vi "Window-Time Series editor.vi"(9 "Standalone viewer?":bool=TRUE) -> ()   [LabVIEW 2020]
uses:
  User Interface/Visualisation/Timelapse Viewer/Typedefs/Custom slider-vertical.ctl
  User Interface/Visualisation/Timelapse Viewer/Typedefs/Time series viewer refs.ctl
  User Interface/Visualisation/Timelapse Viewer/Typedefs/Speed Viewer States enum.ctl
  <vilib>/Utility/miscctls.llb/LVPointTypeDef.ctl
  Typedefs/Save-Load enum.ctl
  <vilib>/vision/Image Controls.llb/IMAQ Image.ctl
  Typedefs/HW config states enum.ctl
  User Interface/Visualisation/Functional Imaging Viewer/Typedefs/Get-Set-Clear Control.ctl
  User Interface/Visualisation/Timelapse Viewer/Typedefs/Select Play-Stop button to show.ctl
  <vilib>/Utility/error.llb/DialogType.ctl
  User Interface/Visualisation/Timelapse Viewer/Cam video sync/Typedefs/Cam videos cluster.ctl
  User Interface/Visualisation/Timelapse Viewer/Globals/gl_Time series viewer globals.vi
  Global Variables/General Globals.vi
panel:
  out "Slider at frame #":i32 format="Slider at frame: %.0f"
  in  "Scrollbar":i32(c297)
  in  "Back":bool
  in  "Play":bool
  in  "Stop":bool
  in  "Tab Control":enum32{"Camera videos", "Speed data"}(tab)
  out "Cams":T2 {"Vid4 Rel time (ms)" format="%.0f ms"; "Vid3 Rel time (ms)" format="%.0f ms"; "Vid2 Rel time (ms)" format="%.0f ms"; "Vid1 Rel time (ms)" format="%.0f ms"}
  out "Actual number of speed points":i32 format="Actual of speed points: %.0f"
  out "Speed Data":string[][](array[string])
  out "Expected speed values":dbl format="Expected speed points: %#_g"
  out "Original frame rate (fps)":dbl format="Original frame rate: %#.1f (fps)"
  out "Frame rate set (fps)":dbl format="Frame rate set: %#.1f (fps)"
  out "Actual frame rate (fps)":dbl format="Actual frame rate: %#.1f (fps)"
  out "AVI Mode ind":string="AVI mode:"
  out "Video length info":string="Duration: 00h 00m 00s, 0 frames"
  in  "AVI File Path":path
  out "Export images":bool
  out "Export snippet":bool
  in  "Selection sliders":cluster{i32, i32}(slide)={1, 5594} scale=1.0..3919.0
  out "Export vid":bool
  out "Stop (ind)":bool
  in  "Intensity":T3={0.0, 4095.0} scale=0.0..4095.0
  in  "Colour":enum16{"Gray", "Red", "Green"}(ring)
  out "Speed Graph":dbl[](graph) caption="Speed Chart"
  out "Image":T1(plugin-control)
  # "Date                         Time                  Time stamp           Speed (rpm)          Angle (deg)"
  # "Time series info"
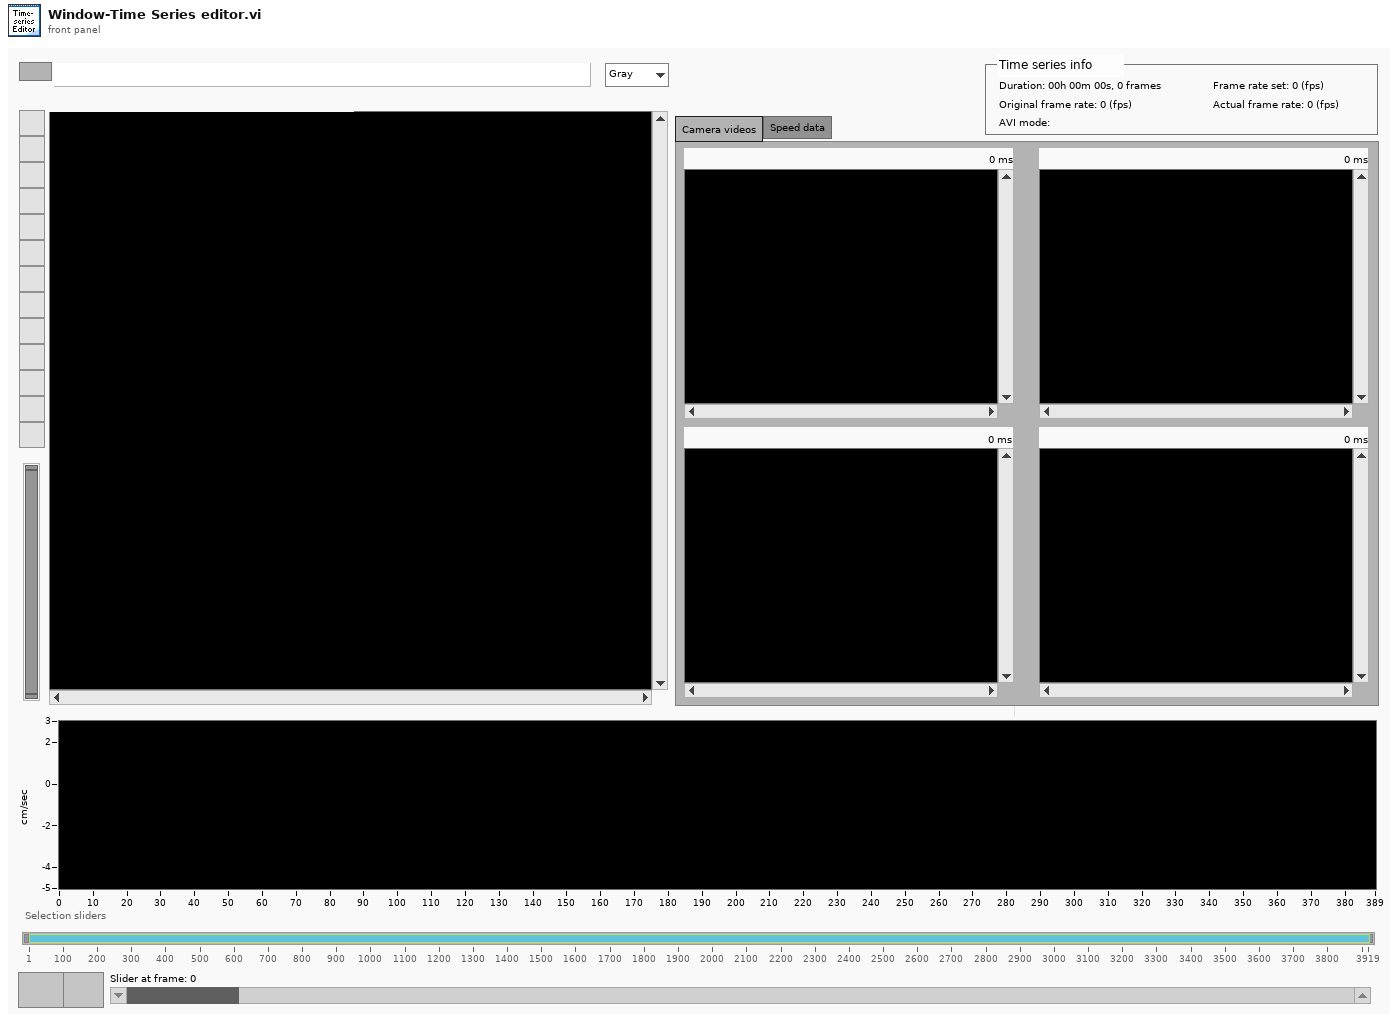
[diagram p1: front panel]
types:
  T1 = typedef "IMAQ Image.ctl" = refnum<image>
  T2 = cluster{"Vid 1":T1, "Vid 2":T1, "Vid 3":T1, "Vid 4":T1, "Vid1 Rel time (ms)":u32, "Vid2 Rel time (ms)":u32, "Vid3 Rel time (ms)":u32, "Vid4 Rel time (ms)":u32}
  T3 = typedef "Custom slider-vertical.ctl" = cluster{dbl, dbl}
  T4 = typedef "Time series viewer refs.ctl" = cluster{"This VI":refnum<vi>, "Image control":refnum<vi>, "AVI Mode ind":refnum<vi>, "Play":refnum<vi>, "Stop":refnum<vi>, "Back":refnum<vi>, "Scrollbar":refnum<vi>, "Video length info":refnum<vi>, "Expected speed values":refnum<vi>, "Intensity":refnum<vi>, "Path":refnum<vi>, "Selection sliders":refnum<vi>, "Speed Graph ref":refnum<vi>, "Frame rate set (fps)":refnum<vi>, "Number of rows to generate":refnum<vi>, "VL Image Array":refnum<vi>, "Image Scrollbar":refnum<vi>, "Channel to load":refnum<vi>, "Colour":refnum<vi>}
  T5 = typedef "Save-Load enum.ctl" = enum16{"Save to file", "Load from file", "Compare from file", "Save Backup"}
  T6 = enum16{"None", "Release queue", "Obtain queue", "Enqueue", "Get status", "Set status"}
  T7 = typedef "LVPointTypeDef.ctl" = cluster{"Horizontal":i16, "Vertical":i16}
  T8 = typedef "Speed Viewer States enum.ctl" = enum16{"Idle", "Initialise", "Playback", "Scroll bar event", "Speed cursor event", "Back to start", "Exit"}
  T9 = typedef "HW config states enum.ctl" = enum16{"Load from file", "Save to file", "Save backup", "Write all", "Read all", "Write XY stage settings", "Write DAQ FPGA settings", "Write Control FPGA settings", "Write Phys Channels", "Write System Config", "Write HW Config", "Save System Config", "Save HW Config", "Clear", "Compare from file"}
  T10 = typedef "Image Type" = u32
  T11 = typedef "Custom slider-horisontal.ctl" = cluster{dbl, dbl}
  T12 = typedef "Get-Set-Clear Control.ctl" = enum16{"Get", "Set", "Clear"}
  T13 = typedef "Select Play-Stop button to show.ctl" = enum16{"Show Play button", "Show Stop button"}
  T14 = typedef "Cam videos cluster.ctl" = cluster{"Vid 1":T1, "Vid 2":T1, "Vid 3":T1, "Vid 4":T1, "Vid1 Rel time (ms)":u32, "Vid2 Rel time (ms)":u32, "Vid3 Rel time (ms)":u32, "Vid4 Rel time (ms)":u32}
  T15 = typedef "DialogType.ctl" = u16
  T16 = typedef "AVI modes refs cluster.ctl" = cluster{"AVI1 ref":T17, "AVI2 refs":T18[], "AVI # frames":u32[]}
  T17 = typedef "AviRefnum.ctl" = refnum<k1>
  T18 = typedef "IMAQ AVI2 Refnum.ctl" = refnum<k20>
  T19 = cluster{"Start Frame No":i32, "End Frame No":i32}
  T20 = typedef "AVI implementation enum.ctl" = enum16{"AVI1", "AVI2"}
  T21 = cluster{"# of frames to export":i32, "Initial frame's owning file":T18, "8-bit AVI file path":path, "Cursors location":cluster{"Number of first frame":i32, "Number of last frame":i32}}
  T22 = enum32{"Invalid", "Standard", "Closed", "Hidden", "Minimized", "Maximized"}
  T23 = typedef "Speed graph behaviour enum.ctl" = enum16{"Scrolling data", "Scrolling cursor"}
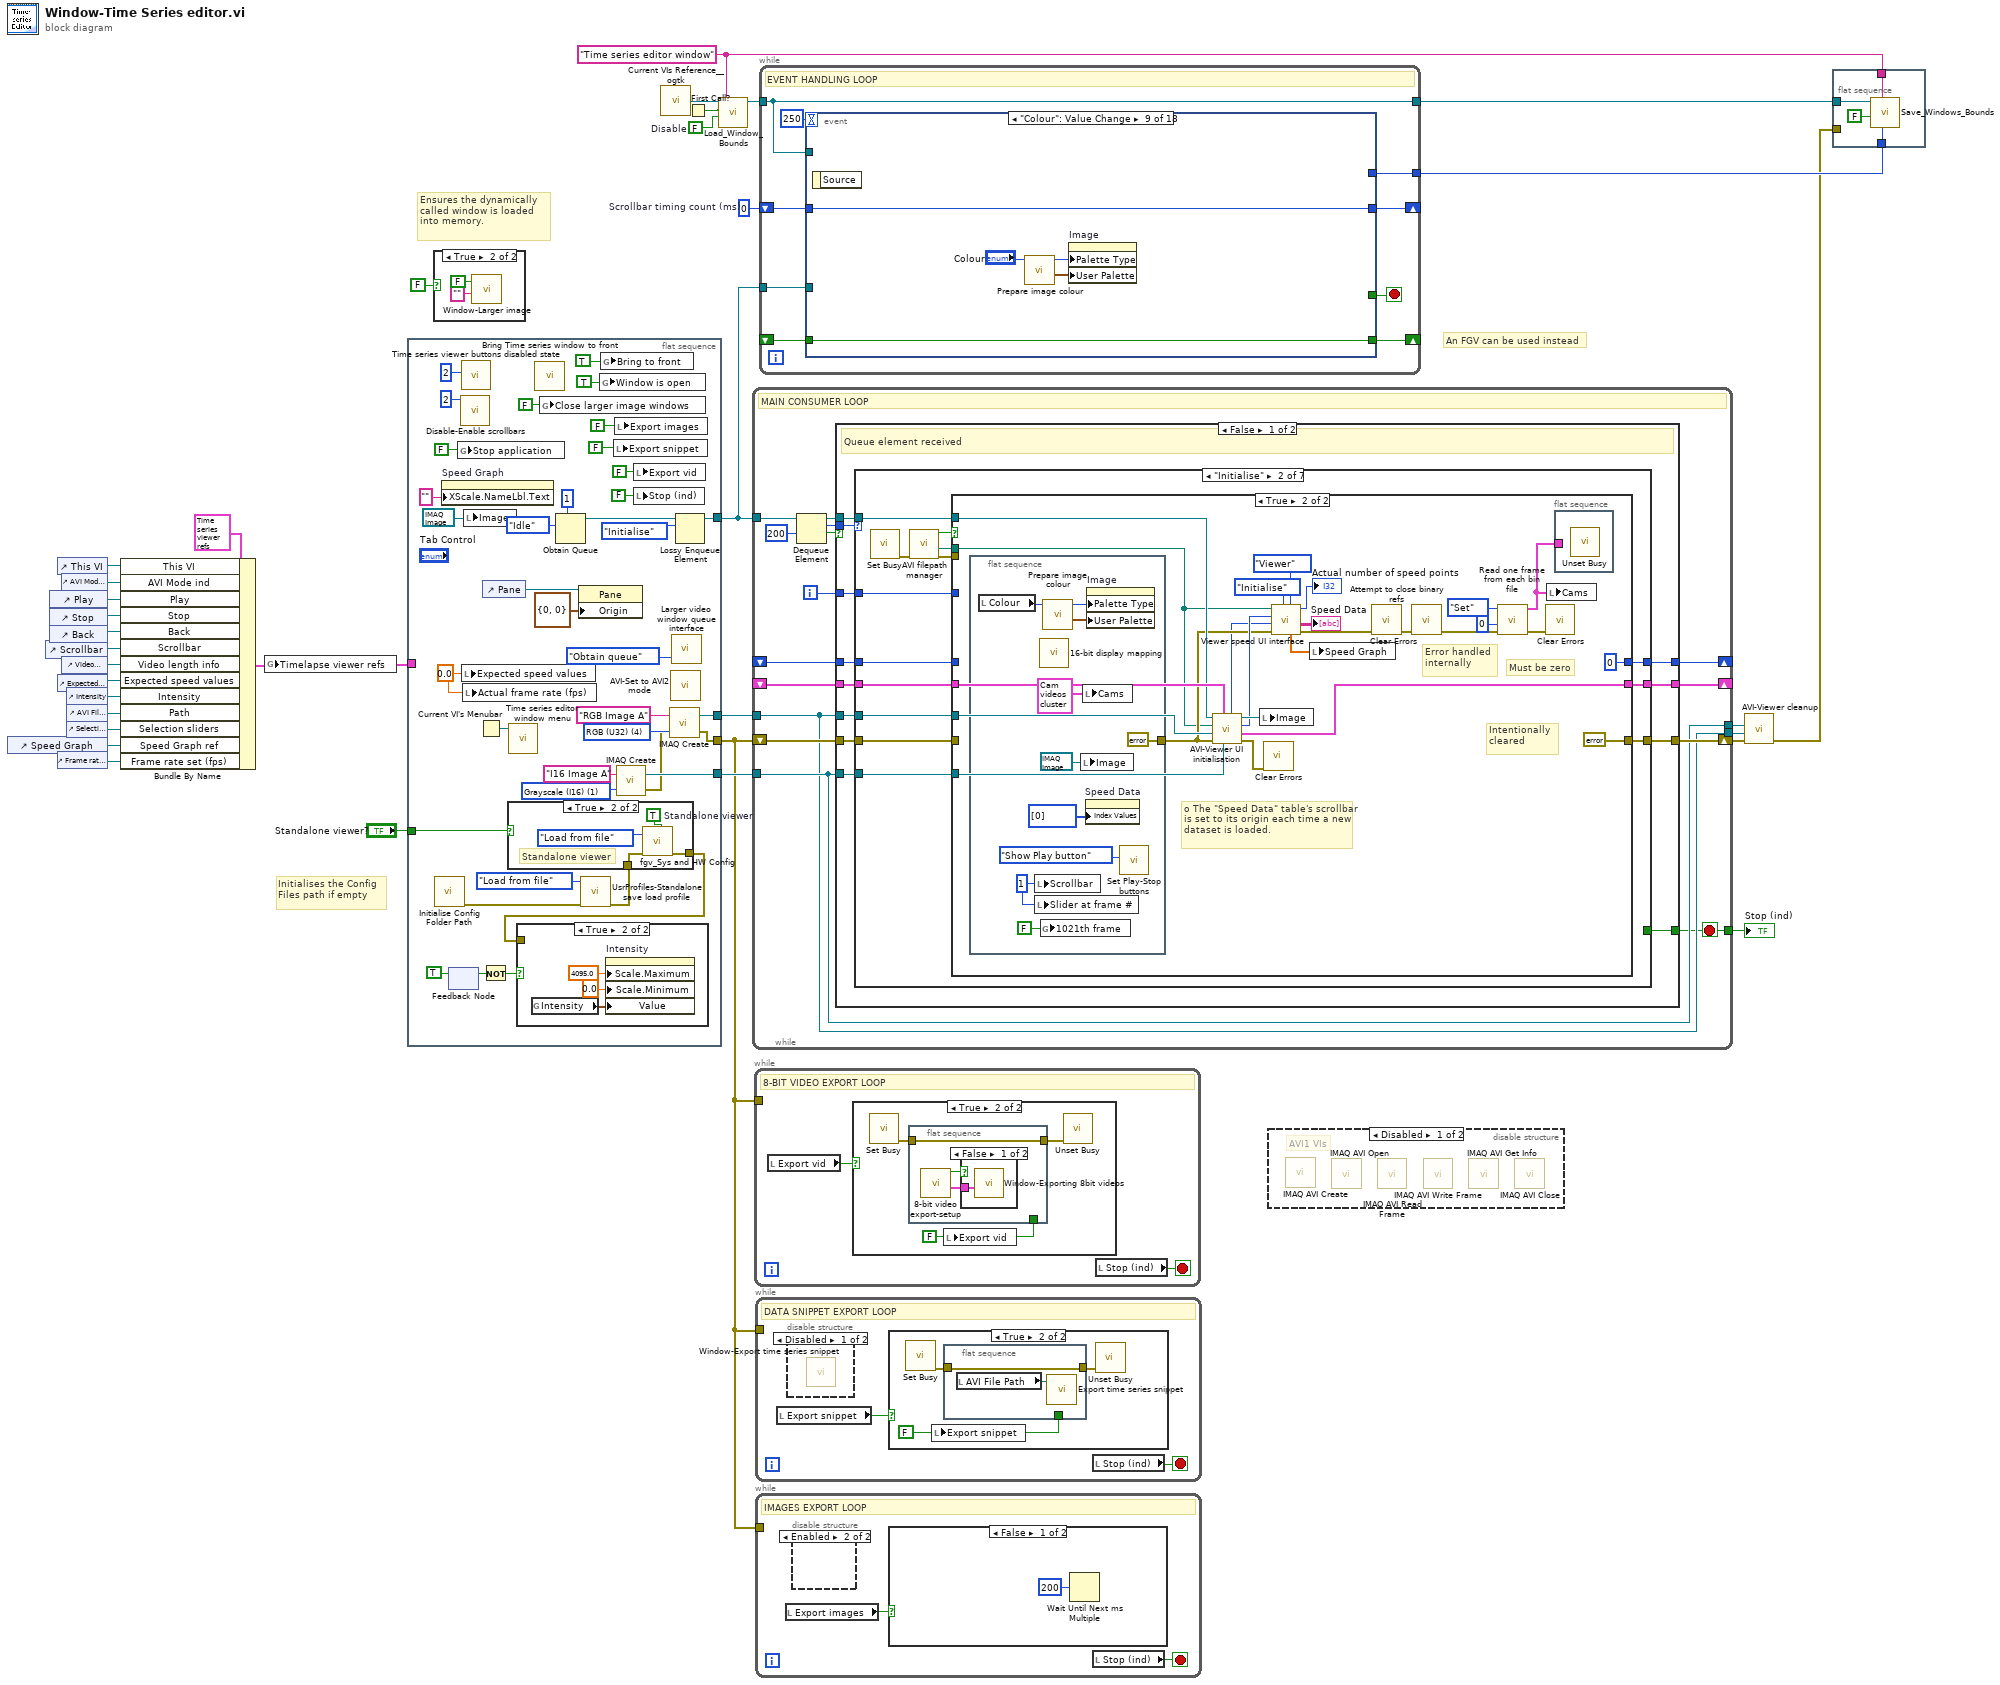
[diagram p0: block diagram]
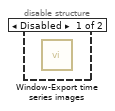
[diagram p3: hidden frame]
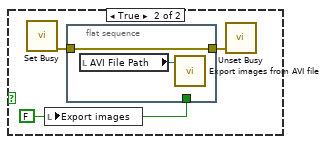
[diagram p4: hidden frame]
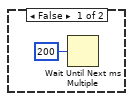
[diagram p6: hidden frame]
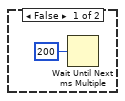
[diagram p8: hidden frame]
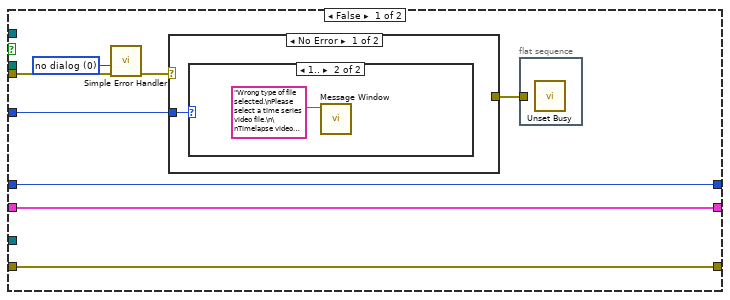
[diagram p13: hidden frame]
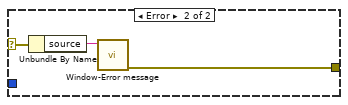
[diagram p15: hidden frame]
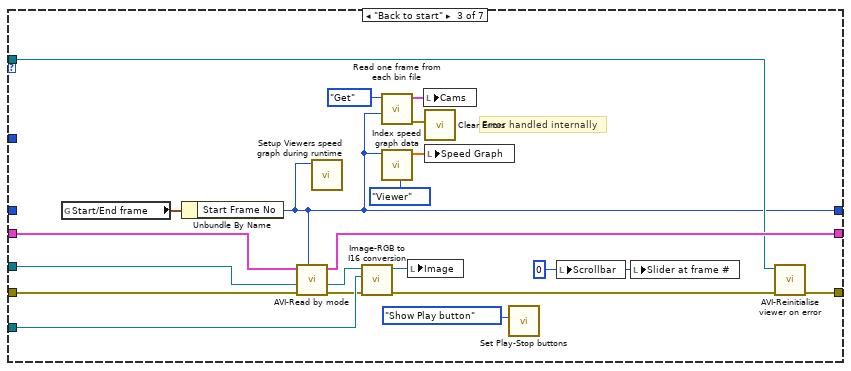
[diagram p16: hidden frame]
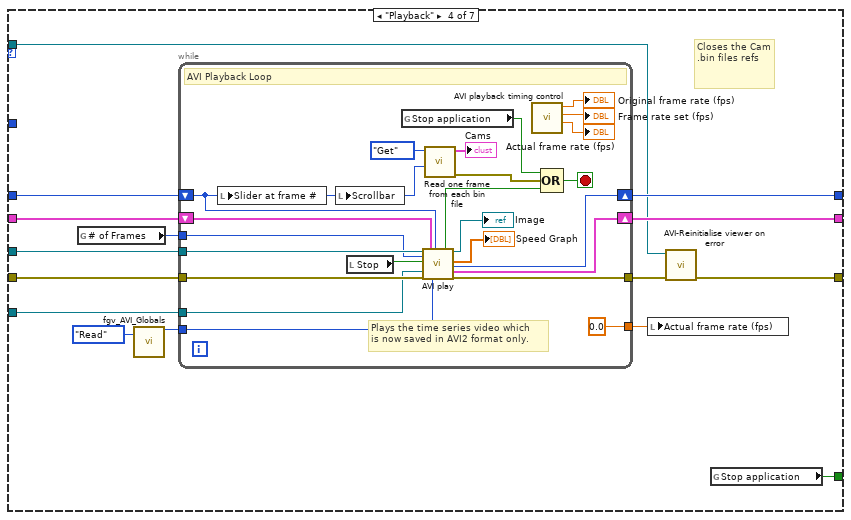
[diagram p17: hidden frame]
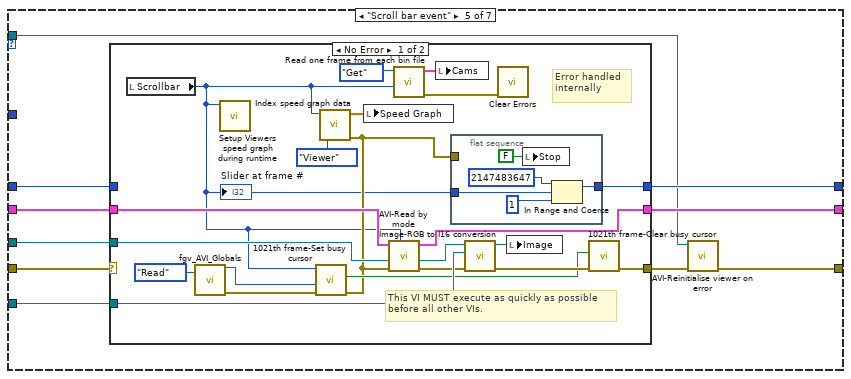
[diagram p18: hidden frame]
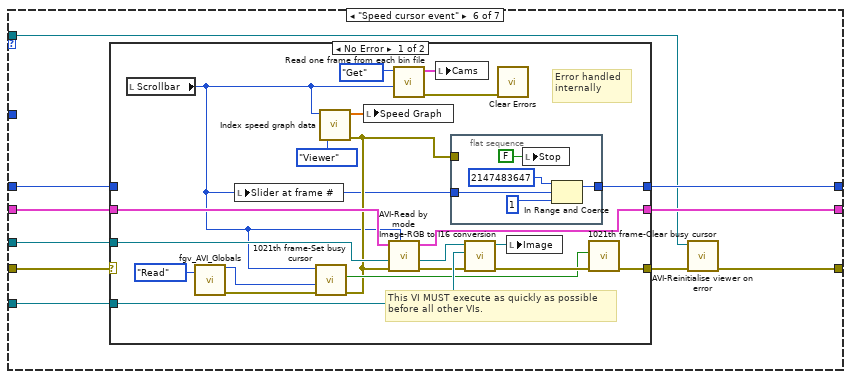
[diagram p20: hidden frame]
diagram:
  w9 = FALSE  # Disable
  w8 = "Time series editor window" ("Window Name (i.e. Key)")
  w20 = u32 0  # Scrollbar timing count (ms)
  # "Initialises the Config Files path if empty"
  # "Ensures the dynamically called window is loaded into memory."
  # "An FGV can be used instead"
  n1 = control-ref of="Speed Graph"() -> (w13:refnum<vi>)
  n2 = control-ref of="Scrollbar"() -> (w24:refnum<vi>)
  n3 = control-ref of="Play"() -> (w27:refnum<vi>)
  n4 = control-ref of="Stop"() -> (w26:refnum<vi>)
  n5 = control-ref of="Back"() -> (w25:refnum<vi>)
  n6 = control-ref of="This VI"() -> (w17:refnum<vi>)
  n7 = control-ref of="Expected speed values"() -> (w22:refnum<vi>)
  n8 = control-ref of="Frame rate set (fps)"() -> (w2:refnum<vi>)
  n9 = control-ref of="AVI Mode ind"() -> (w30:refnum<vi>)
  n10 = control-ref of="Video length info"() -> (w23:refnum<vi>)
  n11 = control-ref of="Intensity"() -> (w21:refnum<vi>)
  n12 = control-ref of="AVI File Path"() -> (w19:refnum<vi>)
  n13 = control-ref of="Selection sliders"() -> (w14:refnum<vi>)
  n14 = Bundle By Name(cluster=T4 {"This VI"=refnum, "Image control"=refnum, "AVI Mode ind"=refnum, "Play"=refnum, "Stop"=refnum, "Back"=refnum, "Scrollbar"=refnum, "Video length info"=refnum, "Expected speed values"=refnum, "Intensity"=refnum, "Path"=refnum, "Selection sliders"=refnum, "Speed Graph ref"=refnum, "Frame rate set (fps)"=refnum, "Number of rows to generate"=refnum, "VL Image Array"=refnum, "Image Scrollbar"=refnum, "Channel to load"=refnum, "Colour"=refnum}, "This VI"=w17, "AVI Mode ind"=w30, "Play"=w27, "Stop"=w26, "Back"=w25, "Scrollbar"=w24, "Video length info"=w23, "Expected speed values"=w22, "Intensity"=w21, "Path"=w19, "Selection sliders"=w14, "Speed Graph ref"=w13, "Frame rate set (fps)"=w2) -> (w16:T4)
  n15 = global write "gl_Time series viewer globals.vi" "Timelapse viewer refs"(w16) -> ()
  n16 = flat-sequence {
    tunnel: [w70] -> w34
    tunnel: [w67] -> w33
    tunnel: [w60] -> w12
    tunnel: [w63] -> w31
    tunnel: w16 -> [_]
    tunnel: "Standalone viewer?" -> [w35]
    frame #0 {
      w57 = 0.0 ("Expected speed points")
      w69 = T10 1 items=["Grayscale (U8)", "Grayscale (I16)", "Grayscale (SGL)", "Complex (CSG)", "RGB (U32)", "HSL (U32)", "RGB (U64)", "Grayscale (U16)"] ("Image Type")
      w71 = T10 4 items=["Grayscale (U8)", "Grayscale (I16)", "Grayscale (SGL)", "Complex (CSG)", "RGB (U32)", "HSL (U32)", "RGB (U64)", "Grayscale (U16)"] ("Image Type")
      n17 = call "Initialise Config Folder Path.vi"() -> ("error out"=w42:errorcluster)  [unwired: 9 in, 2 out]
      n18 = property on="Speed Graph" class="WFGraph (strict)"("XScale.NameLbl.Text"="" ("X Scale.Name Label.Text")) -> ()  [unwired: 2 in, 2 out]
      n19 = feedback #1() -> (w38:bool)  [unwired: 1 in]
      n20 = feedback-in #1(TRUE) -> ()
      n21 = global write "General Globals.vi" "Stop application"(FALSE ("Stop application")) -> ()
      n22 = call "Disable-Enable scrollbars.vi"("Disabled state"=2) -> ()  [unwired: 10 in, 1 out]
      n23 = call "Time series viewer buttons disabled state.vi"("Disabled"=2) -> ()  [unwired: 10 in, 1 out]
      n24 = local write "Expected speed values"(w57) -> ()
      n25 = local write "Actual frame rate (fps)"(w57) -> ()
      n26 = local write "Image"(T1 refnum ("Image")) -> ()
      n27 = Current VI's Menubar() -> (w56:refnum<k9>)
      n28 = Not(x=w38) -> (.not. x?=w40:bool)
      n29 = control-ref of="Pane"() -> (w58:refnum<vi>)
      n30 = call "Time series editor window menu.vi"("menu"=w56) -> ()  [unwired: 9 in, 2 out]
      n31 = call "Bring Time series window to front.vi"() -> ()  [unwired: 12 in]
      n32 = global write "gl_Time series viewer globals.vi" "Close larger image windows"(FALSE ("Close larger image window")) -> ()
      n33 = Obtain Queue(max queue size (-1, unlimited)=1, element data type=Speed_Viewer_States_enum."Idle" ("States")) -> (queue out=w64:refnum<queue>)  [unwired: 3 in, 2 out]
      n34 = property class="Pane"(reference=w58, "Origin"=T7 {"Horizontal"=0, "Vertical"=0}) -> ()  [unwired: 1 in, 2 out]
      n35 = call "UsrProfiles-Standalone save load profile.vi"("Error in"=w42, "Function"=Save-Load_enum."Load from file") -> ("error out"=w37:errorcluster)  [unwired: 9 in]
      n36 = case shown="True" w35 {
        tunnel: w37 -> [w73 w76]
        tunnel: [w73 w75] -> w36
        frame False {
          # "No need to load the system\nconfig. Already loaded."
        }
        frame True {
          w74 = TRUE  # Standalone viewer
          # "Standalone viewer"
          n37 = call "fgv_Sys and HW Config.vi"("Standalone viewer initialisation?"=w74, "Function"=HW_config_states_enum."Load from file", "error in (no error)"=w76) -> ("error out"=w75:errorcluster)  [unwired: 6 in, 2 out]
        }
      }
      n38 = case shown="True" w40 {
        tunnel: w36 -> [_ _]
        frame False {
        }
        frame True {
          n39 = global read "gl_Time series viewer globals.vi" "Intensity"() -> (w78:T11)
          n40 = property on="Intensity" class="Slide (strict)"("Scale.Maximum"=4095.0 ("Scale.Range:Maximum"), "Scale.Minimum"=0.0 ("Scale.Range:Minimum"), "Value"=w78) -> ()  [unwired: 2 in, 2 out]
        }
      }
      n41 = global write "gl_Time series viewer globals.vi" "Window is open"(TRUE ("Window is open")) -> ()
      n42 = global write "gl_Time series viewer globals.vi" "Bring to front"(TRUE ("Bring Timelapse Editor to front")) -> ()
      n43 = local write "Export snippet"(FALSE ("Export data subset")) -> ()
      n44 = local write "Export images"(FALSE ("Export data subset")) -> ()
      n45 = call "IMAQ Create"("Image Name"="I16 Image A", "Image Type"=w69) -> ("New Image"=w67:T1, "error out"=w61:errorcluster)  [unwired: 2 in, 1 out]
      n46 = local write "Export vid"(FALSE ("Export")) -> ()
      n47 = local write "Stop (ind)"(FALSE ("Boolean")) -> ()
      n48 = call "IMAQ Create"("Image Name"="RGB Image A", "Image Type"=w71, "error in (no error)"=w61) -> ("New Image"=w70:T1, "error out"=w60:errorcluster)  [unwired: 1 in, 1 out]
      n49 = call "AVI-Set to AVI2 mode.vi"() -> ()  [unwired: 11 in, 1 out]
      n50 = call "Larger video window queue interface.vi"("Function"=T6."Obtain queue") -> ()  [unwired: 10 in, 1 out]
      n51 = Lossy Enqueue Element(queue=w64, element=Speed_Viewer_States_enum."Initialise" ("States")) -> (queue out=w63:refnum<queue>)  [unwired: 1 in, 3 out]
    }
  }
  n52 = case shown="True" FALSE {
    frame False {
    }
    frame True {
      n53 = call "Window-Larger image.vi"("Image name"="", "Open maximised"=FALSE) -> ()  [unwired: 10 in]
    }
  }
  n54 = call <userlib>:"Current VIs Reference__ogtk.vi"() -> ("Current VI's reference"=w11:refnum<vi>)  [unwired: 5 in]
  n55 = First Call?() -> (First Call?: T/F=w10:bool)
  n56 = call "Load_Window_Bounds.vi"("Window Name (i.e. Key)"=w8, "Disable"=w9, "First Call"=w10, "Window VI's Ref"=w11) -> ("reference out"=w5:refnum<vi>)  [unwired: 4 in, 3 out]
  n57 = while {
    tunnel: w34 -> [w86]
    tunnel: w33 -> [w87]
    tunnel: [w87] -> w32
    shift-right: [w94] -> _
    shift-left: _ -> [w93]
    tunnel: w31 -> [w92]
    shift-right: [w88] -> _
    shift-left: _ -> [w97]
    tunnel: [w86] -> w18
    shift-right: [w95] -> w28
    shift-left: w12 -> [w96]
    tunnel: [w84] -> w15
    i -> [w83]
    stop <- w84 stop-if-true
    # "MAIN CONSUMER LOOP"
    n58 = Dequeue Element(queue=w92, timeout in ms (-1)=200) -> (queue out=w85:refnum<queue>, element=w89:T8, timed out?=w90:bool)  [unwired: 1 in, 1 out]
    n59 = case shown="False" w90 {
      tunnel: w97 -> [w109 w321]
      tunnel: [w108 w321] -> w88
      tunnel: w86 -> [w107 _]
      tunnel: w87 -> [w106 _]
      tunnel: w96 -> [w105 w320]
      tunnel: [w104 w320] -> w95
      tunnel: [w103 w322] -> w94
      tunnel: w93 -> [w102 w322]
      tunnel: w89 -> [w101 _]
      tunnel: [w100 w319] -> w84
      tunnel: w85 -> [w99 _]
      tunnel: w83 -> [w98 _]
      frame False {
        # "Queue element received"
        n60 = case shown="\"Initialise\"" w101 {
          tunnel: w109 -> [w111 w126 w192 w209 w238 w277 w313]
          tunnel: [w111 w122 w191 w203 w240 w279 w313] -> w108
          tunnel: w107 -> [_ w121 w189 w208 w239 w278 _]
          tunnel: w106 -> [_ w120 w190 w207 w242 w281 _]
          tunnel: w105 -> [w110 w124 w187 w206 w237 w276 w312]
          tunnel: [w110 w123 w182 w202 w235 w274 w311] -> w104
          tunnel: [w112 w125 w175 w205 w241 w280 1 ("Slide")] -> w103
          tunnel: w102 -> [w112 w119 _ w204 w236 w275 _]
          tunnel: [_ _ _ w195 _ _ TRUE] -> w100
          tunnel: w99 -> [_ w115 w181 w200 w233 w272 _]
          tunnel: w98 -> [_ w114 _ _ _ _ _]
          frame Default {
          }
          frame "Initialise" {
            n61 = call <vilib>:"Set Busy.vi"() -> ("error out"=w113:errorcluster)  [unwired: 10 in, 1 out]
            n62 = call "AVI filepath manager.vi"("error in (no error)"=w113) -> ("error"=w116:errorcluster, "AVI File Path"=w117:path, "File path OK"=w118:bool)  [unwired: 8 in]
            n63 = case shown="True" w118 {
              tunnel: w126 -> [w133 w164]
              tunnel: [w134 0 ("Slide")] -> w125
              tunnel: w117 -> [_ w148]
              tunnel: w124 -> [w132 _]
              tunnel: [w132 errorcluster {"status"=FALSE, "code"=0, "source"=""} ("error out")] -> w123
              tunnel: [w133 w157] -> w122
              tunnel: w121 -> [_ w156]
              tunnel: w120 -> [_ w162]
              tunnel: w119 -> [w134 _]
              tunnel: w116 -> [w131 _]
              tunnel: w115 -> [_ w160]
              tunnel: w114 -> [w128 _]
              frame False {
                w130 = T15 0 items=["no dialog", "OK message", "continue or stop message", "OK message + warnings", "continue/stop + warnings"] ("type of dialog (OK msg:1)")
                n64 = call <vilib>:"Simple Error Handler.vi"("type of dialog (OK msg:1)"=w130, "error in (no error)"=w131) -> ("error out"=w129:errorcluster)  [unwired: 3 in, 4 out]
                n65 = case shown="No Error" w129 {
                  selector: w129 -> [_ w139]
                  tunnel: w128 -> [w135 _]
                  tunnel: [_ w137] -> w127
                  frame No Error {
                    n66 = case shown="1.." w135 {
                      frame 0, Default {
                      }
                      frame 1.. {
                        n67 = call "Message Window.vi"("Message string"="Wrong type of file selected.\nPlease select a time series video file.\n\nTimelapse video files are located  in time series folders \ne.g. \"TimeLapse 02_10_2014 20-22-02\"\nand their file names are similar to this: \"Green Channel 1\"\n\nNote: For time series video files which are part of a split-files sequence e.g. Green Channel 1, Green Channel 2, Green Channel 3... \ndouble click on any one file. The full sequence will open in the viewer regardless of which file you select.") -> ()  [unwired: 10 in, 1 out]
                      }
                    }
                  }
                  frame Error {
                    n68 = Unbundle By Name(w139) -> ("source"=w138:string)
                    n69 = call "Window-Error message.vi"("Message"=w138) -> ("Error Out (no error)"=w137:errorcluster)  [unwired: 10 in]
                  }
                }
                n70 = flat-sequence {
                  tunnel: w127 -> [_]
                  frame #0 {
                    n71 = call <vilib>:"Unset Busy.vi"() -> ()  [unwired: 11 in, 1 out]
                  }
                }
              }
              frame True {
                # "Must be zero"
                # "o\tThe \"Speed Data\" table's scrollbar is set to its origin each time a new dataset is loaded."
                # "Error handled internally"
                # "Intentionally cleared"
                n72 = flat-sequence {
                  tunnel: [errorcluster {"status"=FALSE, "code"=0, "source"=""} ("error out")] -> w149
                  frame #0 {
                    w166 = 1 ("Scrollbar")
                    n73 = local read "Colour"() -> (w171:enum16{"Gray", "Red", "Green"})
                    n74 = local write "Scrollbar"(w166) -> ()
                    n75 = local write "Slider at frame #"(w166) -> ()
                    n76 = call "16-bit display mapping.vi"() -> ()  [unwired: 11 in, 1 out]
                    n77 = global write "gl_Time series viewer globals.vi" "1021th frame"(FALSE ("1021th frame")) -> ()
                    n78 = call "Prepare image colour.vi"("Left Image Palette"=w171) -> ("Color Palette"=w169:cluster{"Red":u8, "Green":u8, "Blue":u8}[], "Palette Type"=w170:u32)  [unwired: 8 in, 1 out]
                    n79 = local write "Image"(T1 refnum ("New Image")) -> ()
                    n80 = local write "Cams"(T14 {"Vid 1"=refnum, "Vid 2"=refnum, "Vid 3"=refnum, "Vid 4"=refnum, "Vid1 Rel time (ms)"=0, "Vid2 Rel time (ms)"=0, "Vid3 Rel time (ms)"=0, "Vid4 Rel time (ms)"=0} ("Cam videos cluster")) -> ()
                    n81 = property on="Speed Data" class="Arr (strict)"("Index Values"=u32[] [0]) -> ()  [unwired: 2 in, 2 out]
                    n82 = property on="Image" class="ImageControl"("Palette Type"=w170, "User Palette"=w169) -> ()  [unwired: 2 in, 2 out]
                    n83 = call "Set Play-Stop buttons.vi"("Function"=Select_Play-Stop_button_to_show."Show Play button") -> ()  [unwired: 10 in, 1 out]
                  }
                }
                n84 = call "AVI-Viewer UI initialisation.vi"("I16 image ref in"=w162, "AVI modes refs in"=w164, "error in (no error)"=w149, "RGB image ref in"=w156, "AVI File Path"=w148, "Queue in"=w160) -> ("error out"=w143:errorcluster, "AVI modes refs out"=w157:T16, "Number of Frames"=w158:u32, "Refnum out"=w159:T1, "Scrollbar position"=w142:i32)  [unwired: 1 in]
                n85 = local write "Image"(w159) -> ()
                n86 = call <vilib>:"Clear Errors.vi"("error in (no error)"=w143) -> ()  [unwired: 5 in, 2 out]
                n87 = call "Viewer speed UI interface.vi"("Caller"=enum16{"Viewer", "Exporter"}."Viewer", "Function"=enum16{"Initialise", "Update"}."Initialise", "error in (no error)"=w149, "Gobal frame number in Timelapse data/master video (1 based)"=w142, "Number of Frames"=w158, "Speed Data folder path+dummy filename"=w148) -> ("error out"=w154:errorcluster, "Speed Data"=→"Speed Data":string[][], "Actual number of speed values"=→"Actual number of speed points":i32, "Speed waveform graph data"=w163:dbl[])  [unwired: 2 in]
                n88 = local write "Speed Graph"(w163) -> ()
                n89 = call <vilib>:"Clear Errors.vi"("error in (no error)"=w154) -> ("error out"=w150:errorcluster)  [unwired: 5 in, 1 out]
                n90 = call "Attempt to close binary refs.vi"("error in (no error)"=w150) -> ("error out"=w151:errorcluster)  [unwired: 10 in]
                n91 = call "Read one frame from each bin file.vi"("error in (no error)"=w151, "Master video's frame number (unity-based)"=0 ("Frame number"), "Get/set"=Get-Set-Clear_Control."Set" ("GEt set .bin refs")) -> ("Error out"=w144:errorcluster, "Cam videos cluster"=w147:T14)  [unwired: 7 in]
                n92 = call <vilib>:"Clear Errors.vi"("error in (no error)"=w144) -> ()  [unwired: 5 in, 2 out]
                n93 = local write "Cams"(w147) -> ()
                n94 = flat-sequence {
                  tunnel: w147 -> [_]
                  frame #0 {
                    n95 = call <vilib>:"Unset Busy.vi"() -> ()  [unwired: 11 in, 1 out]
                  }
                }
              }
            }
          }
          frame "Back to start" {
            w194 = 0 ("Scrollbar")
            # "Error handled internally"
            n96 = global read "gl_Time series viewer globals.vi" "Start/End frame"() -> (w176:T19)
            n97 = Unbundle By Name(w176) -> ("Start Frame No"=w175:i32)
            n98 = call "AVI-Read by mode.vi"("Frame number (unity-based)"=w175, "error in (no error)"=w187, "RGB image ref in"=w189, "AVI modes refs"=w192) -> ("error out"=w186:errorcluster, "RGB image ref out"=w193:T1, "AVI modes refs"=w191:T16)  [unwired: 5 in]
            n99 = call "Setup Viewers speed graph during runtime.vi"("Frame number or cycle number"=w175) -> ()  [unwired: 10 in, 1 out]
            n100 = call "Image-RGB to I16 conversion.vi"("error in (no error)"=w186, "I16 image ref in"=w190, "RGB image ref in"=w193) -> ("error out"=w183:errorcluster, "I16 image ref out"=w188:T1)  [unwired: 7 in]
            n101 = call "Read one frame from each bin file.vi"("Master video's frame number (unity-based)"=w175, "Get/set"=Get-Set-Clear_Control."Get" ("GEt set .bin refs")) -> ("Error out"=w178:errorcluster, "Cam videos cluster"=w180:T14)  [unwired: 8 in]
            n102 = call "Index speed graph data.vi"("Caller"=enum16{"Viewer", "Exporter"}."Viewer", "Gobal frame number in Timelapse data/master video (1 based)"=w175) -> ("Speed data waveform graph"=w184:dbl[])  [unwired: 7 in, 2 out]
            n103 = local write "Image"(w188) -> ()
            n104 = local write "Cams"(w180) -> ()
            n105 = call <vilib>:"Clear Errors.vi"("error in (no error)"=w178) -> ()  [unwired: 5 in, 2 out]
            n106 = local write "Speed Graph"(w184) -> ()
            n107 = call "Set Play-Stop buttons.vi"("Function"=Select_Play-Stop_button_to_show."Show Play button") -> ()  [unwired: 10 in, 1 out]
            n108 = local write "Scrollbar"(w194) -> ()
            n109 = local write "Slider at frame #"(w194) -> ()
            n110 = call "AVI-Reinitialise viewer on error.vi"("error in (no error)"=w183, "Queue in"=w181) -> ("error out"=w182:errorcluster)  [unwired: 9 in]
          }
          frame "Playback" {
            # "Closes the Cam .bin files refs"
            n111 = global read "gl_Time series viewer globals.vi" "# of Frames"() -> (w197:u32)
            n112 = call "fgv_AVI_Globals.vi"("Function"=enum16{"Intialize", "Write", "Read", "Clear"}."Read") -> ("AVI mode"=w198:T20)  [unwired: 11 in, 3 out]
            n113 = while {
              tunnel: w208 -> [w230]
              tunnel: w207 -> [w220]
              tunnel: w206 -> [w228]
              tunnel: [w229] -> w201
              shift-right: [w226] -> w205
              shift-left: w204 -> [w215]
              shift-right: [w231] -> w203
              shift-left: w209 -> [w232]
              tunnel: w198 -> [w222]
              tunnel: w197 -> [w219]
              tunnel: [0.0 ("Expected speed points")] -> w196
              stop <- w212 stop-if-true
              # "Plays the time series video which \nis now saved in AVI2 format only."
              # "AVI Playback Loop"
              n114 = local write "Slider at frame #"(w215) -> ()
              n115 = local write "Scrollbar"(w215) -> ()
              n116 = local read "Stop"() -> (w221:bool)
              n117 = global read "General Globals.vi" "Stop application"() -> (w210:bool)
              n118 = call "AVI play.vi"("RGB Image ref"=w230, "Number of Frames"=w219, "Stop button pressed"=w221, "I16 Image ref"=w220, "error in (no error)"=w228, "AVI modes refs in"=w232, "AVI mode"=w222, "Frame number (in)"=w215) -> ("Playback stopped"=w213:bool, "I16 image ref out"=→"Image":T1, "Speed data waveform graph"=→"Speed Graph":dbl[], "Frame number (out)"=w226:i32, "AVI modes refs out"=w231:T16, "error out"=w229:errorcluster)  [unwired: 6 in]
              n119 = call "Read one frame from each bin file.vi"("Master video's frame number (unity-based)"=w215, "Get/set"=Get-Set-Clear_Control."Get" ("GEt set .bin refs")) -> ("Error out"=w211:errorcluster, "Cam videos cluster"=→"Cams":T14)  [unwired: 8 in]
              n120 = call "AVI playback timing control.vi"() -> ("Actual frame rate (fps)"=→"Actual frame rate (fps)":dbl, "Frame rate set OR original (fps)"=→"Frame rate set (fps)":dbl, "Original frame rate (fps)"=→"Original frame rate (fps)":dbl)  [unwired: 8 in, 1 out]
              n121 = Compound Arithmetic op=OR(w210, w211, w213) -> (w212:bool)
            }
            n122 = local write "Actual frame rate (fps)"(w196) -> ()
            n123 = call "AVI-Reinitialise viewer on error.vi"("error in (no error)"=w201, "Queue in"=w200) -> ("error out"=w202:errorcluster)  [unwired: 9 in]
            n124 = global read "General Globals.vi" "Stop application"() -> (w195:bool)
          }
          frame "Scroll bar event" {
            n125 = case shown="No Error" w237 {
              selector: w237 -> [_ w271]
              tunnel: w242 -> [w263 _]
              tunnel: [w261 w270] -> w241
              tunnel: [w250 w269] -> w240
              tunnel: w239 -> [w259 _]
              tunnel: w238 -> [w257 w269]
              tunnel: [w252 w271] -> w234
              tunnel: w236 -> [_ w270]
              frame No Error {
                # "Error handled internally"
                # "This VI MUST execute as quickly as possible\nbefore all other VIs."
                n126 = local read "Scrollbar"() -> (w243:i32)
                "Slider at frame #" <- w243
                n127 = call "fgv_AVI_Globals.vi"("Function"=enum16{"Intialize", "Write", "Read", "Clear"}."Read") -> ("AVI mode"=w255:T20, "error out"=w254:errorcluster)  [unwired: 11 in, 2 out]
                n128 = call "Setup Viewers speed graph during runtime.vi"("Frame number or cycle number"=w243) -> ()  [unwired: 10 in, 1 out]
                n129 = call "1021th frame-Set busy cursor.vi"("error in (no error)"=w254, "AVI mode"=w255, "Frame number"=w243) -> ("error out"=w245:errorcluster, "Busy cursor was set"=w251:bool)  [unwired: 7 in]
                n130 = call "Index speed graph data.vi"("Caller"=enum16{"Viewer", "Exporter"}."Viewer", "error in (no error)"=w245, "Gobal frame number in Timelapse data/master video (1 based)"=w243) -> ("Speed data waveform graph"=w246:dbl[])  [unwired: 6 in, 2 out]
                n131 = local write "Speed Graph"(w246) -> ()
                n132 = call "AVI-Read by mode.vi"("Frame number (unity-based)"=w243, "error in (no error)"=w245, "RGB image ref in"=w259, "AVI modes refs"=w257) -> ("error out"=w260:errorcluster, "RGB image ref out"=w258:T1, "AVI modes refs"=w250:T16)  [unwired: 5 in]
                n133 = call "Read one frame from each bin file.vi"("Master video's frame number (unity-based)"=w243, "Get/set"=Get-Set-Clear_Control."Get" ("GEt set .bin refs")) -> ("Error out"=w247:errorcluster, "Cam videos cluster"=w249:T14)  [unwired: 8 in]
                n134 = local write "Cams"(w249) -> ()
                n135 = flat-sequence {
                  tunnel: [w266] -> w261
                  tunnel: w243 -> [w264]
                  tunnel: w245 -> [_]
                  frame #0 {
                    n136 = local write "Stop"(FALSE ("Stop")) -> ()
                    n137 = In Range and Coerce(upper limit=2147483647, x=w264, lower limit=1) -> (coerced(x)=w266:i32)  [unwired: 1 out]
                  }
                }
                n138 = call "Image-RGB to I16 conversion.vi"("error in (no error)"=w260, "I16 image ref in"=w263, "RGB image ref in"=w258) -> ("error out"=w253:errorcluster, "I16 image ref out"=w262:T1)  [unwired: 7 in]
                n139 = call <vilib>:"Clear Errors.vi"("error in (no error)"=w247) -> ()  [unwired: 5 in, 2 out]
                n140 = local write "Image"(w262) -> ()
                n141 = call "1021th frame-Clear busy cursor.vi"("error in (no error)"=w253, "Busy cursor was set"=w251) -> ("error out"=w252:errorcluster)  [unwired: 9 in]
              }
              frame Error {
              }
            }
            n142 = call "AVI-Reinitialise viewer on error.vi"("error in (no error)"=w234, "Queue in"=w233) -> ("error out"=w235:errorcluster)  [unwired: 9 in]
          }
          frame "Speed cursor event" {
            n143 = case shown="No Error" w276 {
              selector: w276 -> [_ w310]
              tunnel: w281 -> [w302 _]
              tunnel: [w300 w309] -> w280
              tunnel: [w289 w308] -> w279
              tunnel: w278 -> [w298 _]
              tunnel: w277 -> [w296 w308]
              tunnel: [w291 w310] -> w273
              tunnel: w275 -> [_ w309]
              frame No Error {
                # "Error handled internally"
                # "This VI MUST execute as quickly as possible\nbefore all other VIs."
                n144 = local read "Scrollbar"() -> (w282:i32)
                n145 = call "fgv_AVI_Globals.vi"("Function"=enum16{"Intialize", "Write", "Read", "Clear"}."Read") -> ("AVI mode"=w294:T20, "error out"=w293:errorcluster)  [unwired: 11 in, 2 out]
                n146 = local write "Slider at frame #"(w282) -> ()
                n147 = call "1021th frame-Set busy cursor.vi"("error in (no error)"=w293, "AVI mode"=w294, "Frame number"=w282) -> ("error out"=w284:errorcluster, "Busy cursor was set"=w290:bool)  [unwired: 7 in]
                n148 = call "Index speed graph data.vi"("Caller"=enum16{"Viewer", "Exporter"}."Viewer", "error in (no error)"=w284, "Gobal frame number in Timelapse data/master video (1 based)"=w282) -> ("Speed data waveform graph"=w285:dbl[])  [unwired: 6 in, 2 out]
                n149 = local write "Speed Graph"(w285) -> ()
                n150 = call "AVI-Read by mode.vi"("Frame number (unity-based)"=w282, "error in (no error)"=w284, "RGB image ref in"=w298, "AVI modes refs"=w296) -> ("error out"=w299:errorcluster, "RGB image ref out"=w297:T1, "AVI modes refs"=w289:T16)  [unwired: 5 in]
                n151 = call "Read one frame from each bin file.vi"("Master video's frame number (unity-based)"=w282, "Get/set"=Get-Set-Clear_Control."Get" ("GEt set .bin refs")) -> ("Error out"=w286:errorcluster, "Cam videos cluster"=w288:T14)  [unwired: 8 in]
                n152 = local write "Cams"(w288) -> ()
                n153 = flat-sequence {
                  tunnel: [w305] -> w300
                  tunnel: w282 -> [w303]
                  tunnel: w284 -> [_]
                  frame #0 {
                    n154 = local write "Stop"(FALSE ("Stop")) -> ()
                    n155 = In Range and Coerce(upper limit=2147483647, x=w303, lower limit=1) -> (coerced(x)=w305:i32)  [unwired: 1 out]
                  }
                }
                n156 = call "Image-RGB to I16 conversion.vi"("error in (no error)"=w299, "I16 image ref in"=w302, "RGB image ref in"=w297) -> ("error out"=w292:errorcluster, "I16 image ref out"=w301:T1)  [unwired: 7 in]
                n157 = call <vilib>:"Clear Errors.vi"("error in (no error)"=w286) -> ()  [unwired: 5 in, 2 out]
                n158 = local write "Image"(w301) -> ()
                n159 = call "1021th frame-Clear busy cursor.vi"("error in (no error)"=w292, "Busy cursor was set"=w290) -> ("error out"=w291:errorcluster)  [unwired: 9 in]
              }
              frame Error {
              }
            }
            n160 = call "AVI-Reinitialise viewer on error.vi"("error in (no error)"=w273, "Queue in"=w272) -> ("error out"=w274:errorcluster)  [unwired: 9 in]
          }
          frame "Exit" {
            n161 = local read "Stop"() -> (w317:bool)
            n162 = Unbundle By Name(w313) -> ("AVI2 refs"=w314:T18[])
            n163 = case shown="True" w317 {
              frame False {
              }
              frame True {
                n164 = local write "Stop"(FALSE ("Stop")) -> ()
              }
            }
            n165 = call "AVI-AVI2 Close all.vi"("error in (no error)"=w312, "AVI2 ref"=w314) -> ("error out"=w311:errorcluster)  [unwired: 9 in]
          }
        }
      }
      frame True {
        # "Timeout"
        n166 = global read "General Globals.vi" "Stop application"() -> (w319:bool)
      }
    }
  }
  "Stop (ind)" <- w15
  n167 = while {
    tunnel: w12 -> [_]
    stop <- w324 stop-if-true
    # "8-BIT VIDEO EXPORT LOOP"
    n168 = local read "Export vid"() -> (w323:bool)
    n169 = case shown="True" w323 {
      frame False {
        n170 = Wait Until Next ms Multiple(millisecond multiple=u32 200) -> ()  [unwired: 1 out]
      }
      frame True {
        w328 = FALSE ("Export")
        n171 = call <vilib>:"Set Busy.vi"() -> ("error out"=w327:errorcluster)  [unwired: 10 in, 1 out]
        n172 = flat-sequence {
          tunnel: w328 -> [_]
          tunnel: w327 -> [w331]
          tunnel: [w331] -> w326
          frame #0 {
            n173 = call "8-bit video export-setup.vi"() -> ("output cluster"=w330:T21, "cancelled"=w329:bool)  [unwired: 9 in, 1 out]
            n174 = case shown="False" w329 {
              tunnel: w330 -> [w332 _]
              frame False {
                n175 = call "Window-Exporting 8bit videos.vi"("Input cluster"=w332) -> ()  [unwired: 11 in]
              }
              frame True {
              }
            }
          }
        }
        n176 = local write "Export vid"(w328) -> ()
        n177 = call <vilib>:"Unset Busy.vi"("error in (no error)"=w326) -> ()  [unwired: 10 in, 1 out]
      }
    }
    n178 = local read "Stop (ind)"() -> (w324:bool)
  }
  n179 = while {
    tunnel: w12 -> [_]
    stop <- w334 stop-if-true
    # "DATA SNIPPET EXPORT LOOP"
    n180 = local read "Export snippet"() -> (w333:bool)
    n181 = disable-structure shown="Disabled" {
      frame Disabled {
        n182 = call "Window-Export time series snippet.vi"() -> ()  [unwired: 12 in]
      }
      frame Enabled {
      }
    }
    n183 = case shown="True" w333 {
      frame False {
        n184 = Wait Until Next ms Multiple(millisecond multiple=u32 200) -> ()  [unwired: 1 out]
      }
      frame True {
        w338 = FALSE ("Export data subset")
        n185 = call <vilib>:"Set Busy.vi"() -> ("error out"=w337:errorcluster)  [unwired: 10 in, 1 out]
        n186 = local write "Export snippet"(w338) -> ()
        n187 = flat-sequence {
          tunnel: w338 -> [_]
          tunnel: w337 -> [w340]
          tunnel: [w340] -> w336
          frame #0 {
            n188 = local read "AVI File Path"() -> (w339:path)
            n189 = call "Export time series snippet.vi"("AVI File Path"=w339) -> ()  [unwired: 11 in]
          }
        }
        n190 = call <vilib>:"Unset Busy.vi"("error in (no error)"=w336) -> ()  [unwired: 10 in, 1 out]
      }
    }
    n191 = local read "Stop (ind)"() -> (w334:bool)
  }
  n192 = while {
    tunnel: w12 -> [_]
    stop <- w342 stop-if-true
    # "IMAGES EXPORT LOOP"
    n193 = local read "Export images"() -> (w341:bool)
    n194 = disable-structure shown="Enabled" {
      frame Disabled {
        n195 = call "Window-Export time series images.vi"() -> ()  [unwired: 12 in]
      }
      frame Enabled {
      }
    }
    n196 = case shown="False" w341 {
      frame False {
        n197 = Wait Until Next ms Multiple(millisecond multiple=u32 200) -> ()  [unwired: 1 out]
      }
      frame True {
        w344 = FALSE ("Export data subset")
        n198 = call <vilib>:"Set Busy.vi"() -> ("error out"=w346:errorcluster)  [unwired: 10 in, 1 out]
        n199 = local write "Export images"(w344) -> ()
        n200 = flat-sequence {
          tunnel: w344 -> [_]
          tunnel: w346 -> [w348]
          tunnel: [w348] -> w345
          frame #0 {
            n201 = local read "AVI File Path"() -> (w347:path)
            n202 = call "Export images from AVI file.vi"("AVI File Path"=w347) -> ()  [unwired: 11 in]
          }
        }
        n203 = call <vilib>:"Unset Busy.vi"("error in (no error)"=w345) -> ()  [unwired: 10 in, 1 out]
      }
    }
    n204 = local read "Stop (ind)"() -> (w342:bool)
  }
  n205 = while {
    shift-right: [w355] -> _
    shift-left: w20 -> [w354]
    tunnel: w31 -> [w353]
    shift-right: [w352] -> _
    shift-left: _ -> [w351]
    tunnel: [w350] -> w4
    tunnel: w5 -> [w349]
    tunnel: [w349] -> w6
    stop <- w356 stop-if-true
    # "EVENT HANDLING LOOP"
    n206 = event shown="[8] \"Colour\": Value Change" {
      selector: _ -> [_ _ _ _ _ _ _ _ _ _ _ _ _ _ _ _ _ _]
      dyn-events: _ -> [_ _ _ _ _ _ _ _ _ _ _ _ _ _ _ _ _ _]
      timeout: 250 -> [_ _ _ _ _ _ _ _ _ _ _ _ _ _ _ _ _ _]
      tunnel: [w358 w364 _ _ _ _ _ _ _ _ _ _ _ _ _ _ _ w488] -> w356
      tunnel: [w362 w367 w378 w382 w391 w397 w405 w418 w432 w436 w443 w451 w456 w461 w464 w466 w483 w490] -> w355
      tunnel: w354 -> [w362 w367 w378 w384 w391 w397 w405 w420 w432 w436 w443 w451 w456 w461 w464 w468 w483 w490]
      tunnel: w353 -> [_ w365 _ w383 _ w398 _ w419 _ w435 _ _ _ w458 _ w472 _ w489]
      tunnel: [w361 w363 w379 w381 w390 w400 w404 w409 w428 w434 w439 FALSE FALSE w457 w463 w469 w482 w487] -> w352
      tunnel: w351 -> [w361 w363 w379 w381 w390 w400 w404 w409 w428 w434 _ w450 _ w457 w463 w469 w482 w487]
      tunnel: [w359 _ _ _ _ _ _ _ _ _ _ _ _ _ _ _ _ w486] -> w350
      tunnel: w349 -> [w360 _ _ _ _ _ _ _ _ _ _ _ _ _ _ _ _ w485]
      event Timeout {
        n207 = event-data() -> ()  [unwired: 1 in, 1 out]
        n208 = call "Bring Time series window to front.vi"() -> ()  [unwired: 12 in]
        n209 = global read "General Globals.vi" "Stop application"() -> (w358:bool)
        n210 = property class="VI"(reference=w360) -> ("FP.State"=w359:T22)  [unwired: 1 in, 2 out]
      }
      event Menu Selection (User) {
        n211 = event-data() -> ("ItemTag"=w366:string)  [unwired: 1 in]
        n212 = case shown="\"Close\"" w366 {
          tunnel: w365 -> [_ w368 _ _ w373 _ _ _]
          tunnel: [_ _ _ _ w372 _ _ _] -> w364
          frame Default {
          }
          frame "Load dataset" {
            n213 = call "Time series viewer-Event handler-Load dataset.vi"("queue"=w368) -> ()  [unwired: 11 in]
          }
          frame "Playback speed..." {
            n214 = call "Window-Playback speed entry.vi"() -> ("Frame rate set (fps)"=w369:dbl)  [unwired: 10 in, 1 out]
            n215 = local write "Frame rate set (fps)"(w369) -> ()
          }
          frame "Original speed (x1)" {
            n216 = flat-sequence {
              frame #0 {
                n217 = global write "gl_Time series viewer globals.vi" "Use manual FPS?"(FALSE ("Use manual FPS?")) -> ()
              }
              frame #1 {
                n218 = call "AVI playback timing control.vi"() -> ("Frame rate set OR original (fps)"=w371:dbl)  [unwired: 8 in, 3 out]
                n219 = local write "Frame rate set (fps)"(w371) -> ()
              }
            }
          }
          frame "Close" {
            n220 = call "Time series viewer-Event handler-Exit.vi"("Queue in"=w373) -> ("Exit"=w372:bool)  [unwired: 10 in]
            n221 = case shown="True" w372 {
              frame False {
              }
              frame True {
                n222 = local write "Stop"(TRUE ("Stop")) -> ()
              }
            }
          }
          frame "Export snippet" {
            "Export snippet" <- TRUE
          }
          frame "Export 8-bit video" {
            "Export vid" <- TRUE
          }
          frame "Export TIFF series" {
            "Export images" <- TRUE
          }
        }
      }
      event "Scrollbar", "Speed Graph": Shortcut Menu Selection (User) {
        n223 = event-data() -> ("ItemTag"=w380:string)  [unwired: 1 in]
        n224 = call "Time series viewer-Shortcut menu handler.vi"("ItemTag"=w380) -> ()  [unwired: 11 in]
      }
      event "Scrollbar": Value Change {
        n225 = event-data() -> ()  [unwired: 1 in, 1 out]
        n226 = call "Event case-Scrollbar value change.vi"("Tick count in"=w384, "Queue in"=w383) -> ("Tick count"=w382:u32)  [unwired: 8 in, 1 out]
      }
      event "Speed Graph": Shortcut Menu Activation? {
        n227 = event-data() -> ("MenuRef"=w387:refnum<k9>)  [unwired: 1 in]
        n228 = call "FGV_Speed graph behaviour-Main viewer.vi"("Function"=Get-Set-Clear_Control."Get") -> ("Speed graph behaviour"=w386:T23)  [unwired: 9 in, 1 out]
        n229 = case shown="\"Scrolling data\", Default" w386 {
          tunnel: [bool[] [FALSE, TRUE] bool[] [TRUE, FALSE]] -> w385
          frame "Scrolling data", Default {
          }
          frame "Scrolling cursor" {
          }
        }
        n230 = for {
          tunnel: string[] ["scrolling cursor", "scrolling data"] -> [w396] mode=indexing
          tunnel: w387 -> [w395]
          tunnel: w385 -> [w394] mode=indexing
          n231 = Set Menu Item Info(6:w394, 7:w396, 11:w395) -> ()  [unwired: 4 in, 2 out]
        }
        n232 = event-data() -> ()  [unwired: 2 in, 1 out]
      }
      event "Speed Graph": Cursor Move; "Speed Graph": Cursor Release {
        n233 = event-data() -> ("CursRef"=w399:refnum<vi>)  [unwired: 1 in]
        n234 = call "Event case-Speed graph cursor moved.vi"("queue in"=w398, "Cursor in"=w399) -> ()  [unwired: 9 in, 1 out]
      }
      event "Speed Graph": event type 3.0.x80000027 {
        n235 = event-data() -> ()  [unwired: 1 in, 1 out]
        n236 = call "FGV_Speed graph behaviour-Main viewer.vi"("Function"=Get-Set-Clear_Control."Get") -> ("Speed graph behaviour"=w402:T23)  [unwired: 9 in, 1 out]
        n237 = case shown="\"Scrolling data\", Default" w402 {
          tunnel: [TRUE FALSE] -> w401
          frame "Scrolling data", Default {
            # "Moving the speed data graph's cursor manually is \nprevented when the mode is \"Scrolling data\"."
          }
          frame "Scrolling cursor" {
            # "Moving the speed data graph's cursor manually is \nallowed when the mode is \"Scrolling cursor\"."
          }
        }
        n238 = event-data("Discard?"=w401) -> ()  [unwired: 1 in, 1 out]
      }
      event "Selection sliders": Value Change {
        # "Do not use the left cursor's change event"
        # "Sets the main slider to the value of the extraction cursor that was moved."
        n239 = event-data() -> ("OldVal"=w417:cluster{i32, i32}, "NewVal"=w410:cluster{i32, i32})  [unwired: 1 in]
        n240 = Not Equal?(x=w417, y=w410) -> (x != y?=w411:cluster{bool, bool})
        n241 = Unbundle(w411) -> (w408:bool)  [unwired: 1 out]
        n242 = Unbundle(w410) -> (w416:i32, w415:i32)
        n243 = Select(t=w415, s=w408, f=w416) -> (s? t:f=w412:i32)
        n244 = flat-sequence {
          tunnel: w419 -> [w423]
          tunnel: w420 -> [w424]
          tunnel: [w424] -> w414
          tunnel: [w423] -> w413
          tunnel: w412 -> [w422]
          tunnel: w408 -> [w421]
          tunnel: [w425] -> w418
          tunnel: w414 -> [w427]
          tunnel: w413 -> [w426]
          frame #0 {
            n245 = call "Sync scrollbars.vi"("Min cursor moved"=w421, "Scrollbar value"=w422) -> ()  [unwired: 9 in, 1 out]
          }
          frame #1 {
            n246 = call "Event case-Scrollbar value change.vi"("Tick count in"=w427, "Queue in"=w426) -> ("Tick count"=w425:u32)  [unwired: 8 in, 1 out]
          }
        }
      }
      event "Colour": Value Change {
        n247 = event-data() -> ()  [unwired: 1 in, 1 out]
        n248 = call "Prepare image colour.vi"("Left Image Palette"="Colour") -> ("Color Palette"=w429:cluster{"Red":u8, "Green":u8, "Blue":u8}[], "Palette Type"=w430:u32)  [unwired: 8 in, 1 out]
        n249 = property on="Image" class="ImageControl"("Palette Type"=w430, "User Palette"=w429) -> ()  [unwired: 2 in, 2 out]
      }
      event "AVI File Path": Value Change {
        w433 = TRUE ("Stop")
        n250 = event-data() -> ()  [unwired: 1 in, 1 out]
        n251 = local write "Stop"(w433) -> ()
        n252 = flat-sequence {
          tunnel: w435 -> [w438]
          tunnel: w433 -> [_]
          frame #0 {
            n253 = Enqueue Element At Opposite End(queue=w438, element=Speed_Viewer_States_enum."Initialise") -> ()  [unwired: 2 in, 3 out]
          }
        }
      }
      event "Cams.Vid 1", "Cams.Vid 2", "Cams.Vid 3", "Cams.Vid 4": Mouse Down {
        # "http://zone.ni.com/reference/en-XX/help/371361K-01/lvhowto/drag_and_drop_programmatic_prepare/"
        # "Detects and registers when the mouse is clicked \nwithin the boundaries of a CamVid display. This allows to generate a \"Drag leave\" event for those displays (in a separate event case / Mouse leave case).\nThis is necessary because the Drag-Leave event does not work for this type of control."
        n254 = event-data() -> ("Button"=w440:u16, "Mods.Double Click"=w442:bool, "CtlRef"=w441:refnum<vi>)  [unwired: 1 in]
        n255 = case shown="True" w442 {
          tunnel: w440 -> [_ w445]
          tunnel: w441 -> [_ w447]
          frame False {
          }
          frame True {
            n256 = property class="ImageControl"(reference=w447) -> ("Label.Text"=w446:string)  [unwired: 1 in, 2 out]
            n257 = call "Open expanded image window.vi"("Button"=w445, "Image name"=w446) -> ()  [unwired: 10 in]
          }
        }
        n258 = case shown="1" w440 {
          tunnel: [_ TRUE] -> w439
          frame 0, Default {
          }
          frame 1 {
          }
        }
      }
      event "Cams.Vid 1", "Cams.Vid 2", "Cams.Vid 3", "Cams.Vid 4": Mouse Leave {
        n259 = event-data() -> ("CtlRef"=w448:refnum<vi>)  [unwired: 1 in]
        n260 = case shown="False" w450 {
          tunnel: w448 -> [_ w454]
          frame False {
          }
          frame True {
            n261 = property class="ImageControl"(reference=w454) -> ("Label.Text"=w452:string)  [unwired: 1 in, 2 out]
            n262 = call "Open expanded image window.vi"("Button"=u16 0, "Image name"=w452) -> ()  [unwired: 10 in]
          }
        }
      }
      event Mouse Up {
        n263 = event-data() -> ()  [unwired: 1 in, 1 out]
      }
      event "Back": Value Change {
        n264 = event-data() -> ()  [unwired: 1 in, 1 out]
        n265 = Enqueue Element At Opposite End(queue=w458, element=Speed_Viewer_States_enum."Back to start") -> ()  [unwired: 2 in, 3 out]
        n266 = local write "Stop"(TRUE ("Stop")) -> ()
      }
      event Value Change {
        n267 = event-data() -> ()  [unwired: 1 in, 1 out]
        n268 = global write "gl_Time series viewer globals.vi" "Intensity"("Intensity") -> ()
        n269 = call "16-bit display mapping.vi"() -> ()  [unwired: 11 in, 1 out]
      }
      event "Play": Value Change {
        n270 = event-data() -> ()  [unwired: 1 in, 1 out]
        n271 = flat-sequence {
          tunnel: w472 -> [w476]
          tunnel: [w476] -> w471
          tunnel: w468 -> [w473]
          tunnel: [w473] -> w467
          tunnel: w471 -> [w478]
          tunnel: [w478] -> w470
          tunnel: w467 -> [w477]
          tunnel: [w477] -> w465
          tunnel: w470 -> [w480]
          tunnel: [w479] -> w466
          tunnel: w465 -> [w479]
          frame #0 {
            n272 = local write "Stop"(FALSE ("Stop")) -> ()
            n273 = call "Set Play-Stop buttons.vi"("Function"=Select_Play-Stop_button_to_show."Show Stop button") -> ()  [unwired: 10 in, 1 out]
          }
          frame #1 {
            n274 = call "Set scrollbar at start.vi"("Queue in"=w478) -> ()  [unwired: 10 in, 1 out]
          }
          frame #2 {
            n275 = Enqueue Element(queue=w480, element=Speed_Viewer_States_enum."Playback" ("States")) -> ()  [unwired: 2 in, 3 out]
          }
        }
      }
      event "Stop": Value Change {
        n276 = event-data() -> ()  [unwired: 1 in, 1 out]
      }
      event Panel Close? {
        # "The panel close is always discarded here because it is closed conditionally in the yellow \"Save Windows Bounds\" vi."
        n277 = event-data() -> ()  [unwired: 1 in, 1 out]
        n278 = call "Time series viewer-Event handler-Exit.vi"("Queue in"=w489) -> ("Exit"=w488:bool)  [unwired: 10 in]
        n279 = case shown="True" w488 {
          frame False {
          }
          frame True {
            n280 = local write "Stop"(TRUE ("Stop")) -> ()
            n281 = global write "gl_Time series viewer globals.vi" "Close larger image windows"(TRUE ("Close larger image window")) -> ()
          }
        }
        n282 = property class="VI"(reference=w485) -> ("FP.State"=w486:T22)  [unwired: 1 in, 2 out]
        n283 = event-data("Discard?"=TRUE) -> ()  [unwired: 1 in, 1 out]
      }
    }
  }
  n284 = disable-structure shown="Disabled" {
    frame Disabled {
      # "AVI1 VIs"
      n285 = call "IMAQ AVI Create"() -> ()  [unwired: 10 in, 2 out]
      n286 = call "IMAQ AVI Open"() -> ()  [unwired: 10 in, 2 out]
      n287 = call "IMAQ AVI Read Frame"() -> ()  [unwired: 8 in, 4 out]
      n288 = call "IMAQ AVI Write Frame"() -> ()  [unwired: 10 in, 2 out]
      n289 = call "IMAQ AVI Get Info"() -> ()  [unwired: 7 in, 5 out]
      n290 = call "IMAQ AVI Close"() -> ()  [unwired: 11 in, 1 out]
    }
    frame Enabled {
    }
  }
  n291 = call "AVI-Viewer cleanup.vi"("error in (no error)"=w28, "RGB image ref"=w18, "I16 image ref"=w32) -> ("error out"=w3:errorcluster)  [unwired: 8 in]
  n292 = flat-sequence {
    tunnel: w8 -> [w496]
    tunnel: w6 -> [w494]
    tunnel: w4 -> [w493]
    tunnel: w3 -> [_]
    frame #0 {
      n293 = call "Save_Windows_Bounds.vi"("FP.State"=w493, "Window Name (i.e. Key)"=w496, "Front Panel Window:Open"=FALSE, "Window VI's Ref"=w494) -> ()  [unwired: 7 in, 1 out]
    }
  }
